vi "Write Teller.vi"(10 "Teller":refnum<class "Teller.lvclass">, 11 "TEMPLATE Msg Input in":refnum<class "TEMPLATE Msg Input.lvclass">) -> (3 "TEMPLATE Msg Input out":refnum<class "TEMPLATE Msg Input.lvclass">)   [LabVIEW 2020, in "_Template.lvlib" / "Templates.lvlib" / "TEMPLATE jettl Msg.lvlib" / "TEMPLATE Msg Input.lvlib" / "TEMPLATE Msg Input.lvclass"]
uses:
  TEMPLATE Msg Input.lvclass
  jettl/jettl/Teller/Teller.lvclass
  TEMPLATE Msg Input.lvclass/TEMPLATE Msg Input.ctl
panel:
  # "This front panel should not be manipulated."
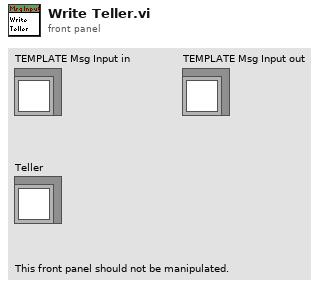
[diagram p1: front panel]
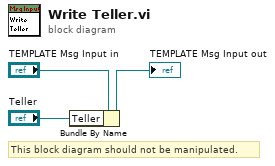
[diagram p0: block diagram]
diagram:
  # "This block diagram should not be manipulated."
  n1 = Bundle By Name(cluster="TEMPLATE Msg Input in", "Teller"="Teller") -> (→"TEMPLATE Msg Input out":refnum<class "TEMPLATE Msg Input.lvclass">)
